vi "Main.vi"(8 "error in (no error)":errorcluster, 11 "Event Registration Refnum":refnum<event-registration>) -> (0 "error out":errorcluster)   [LabVIEW 2023, in "Controller.lvlib"]
uses:
  Controller.lvlib
  Type Def/Module Data.ctl
panel:
  in  "stop":bool
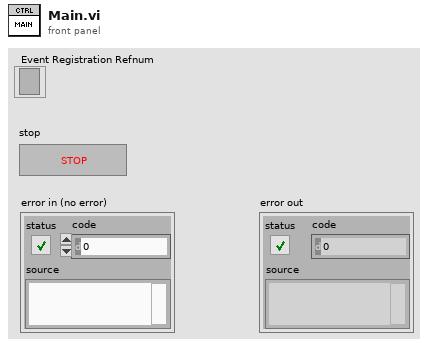
[diagram p1: front panel]
types:
  T1 = typedef "Controller.lvlib/Module Data.ctl" = cluster{"Module Name":string}
  T2 = typedef "Controller.lvlib/Message Data.ctl" = cluster{"Message":string, "Data":variant}
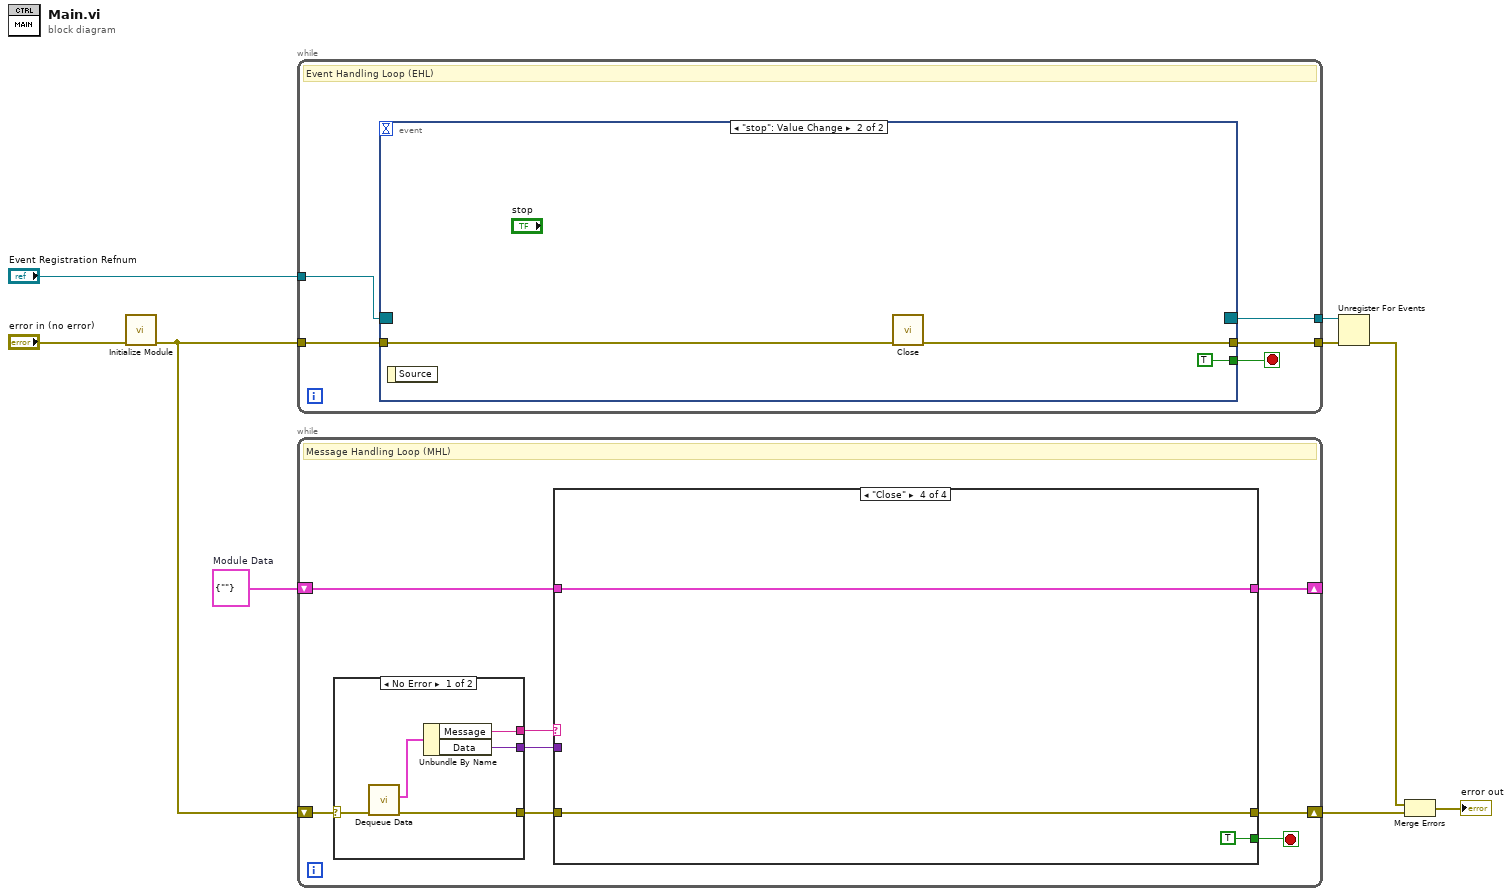
[diagram p0: block diagram]
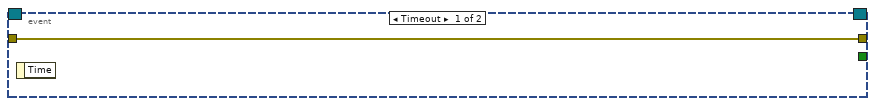
[diagram p2: hidden frame]
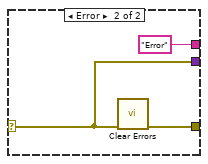
[diagram p3: hidden frame]
diagram:
  w8 = T1 {"Module Name"=""}  # Module Data
  n1 = call "Initialize Module.vi"("error in (no error)"="error in (no error)") -> ("error out"=w7:errorcluster)  [unwired: 10 in]
  n2 = while {
    tunnel: w7 -> [w14]
    tunnel: [w13] -> w4
    tunnel: [w12] -> w2
    tunnel: "Event Registration Refnum" -> [w10]
    stop <- w11 stop-if-true
    # "Event Handling Loop (EHL)"
    n3 = event shown="[1] \"stop\": Value Change" {
      selector: w10 -> [_ _]
      dyn-events: [_ _] -> w12
      timeout: _ -> [_ _]
      tunnel: w14 -> [w15 w18]
      tunnel: [w15 w17] -> w13
      tunnel: [_ TRUE] -> w11
      event Timeout {
        n4 = event-data() -> ()  [unwired: 1 in, 1 out]
      }
      event "stop": Value Change {
        n5 = event-data() -> ()  [unwired: 1 in, 1 out]
        n6 = call "Close.vi"("error in (no error)"=w18) -> ("error out"=w17:errorcluster)  [unwired: 10 in]
      }
    }
  }
  n7 = while {
    shift-right: [w25] -> _
    shift-left: w8 -> [w26]
    shift-right: [w20] -> w6
    shift-left: w7 -> [w24]
    stop <- w19 stop-if-true
    # "Message Handling Loop (MHL)"
    n8 = case shown="No Error" w24 {
      selector: w24 -> [w31 w32]
      tunnel: [w29 "Error" ("Message")] -> w23
      tunnel: [w28 w32] -> w22
      tunnel: [w27 w33] -> w21
      frame No Error {
        n9 = call "Dequeue Data.vi"("error in (no error)"=w31) -> ("error out"=w27:errorcluster, "Message Data"=w30:T2)  [unwired: 9 in]
        n10 = Unbundle By Name(w30) -> ("Message"=w29:string, "Data"=w28:variant)
      }
      frame Error {
        n11 = call <vilib>:"Clear Errors.vi"("error in (no error)"=w32) -> ("error out"=w33:errorcluster)  [unwired: 5 in, 1 out]
      }
    }
    n12 = case shown="\"Close\"" w23 {
      tunnel: w26 -> [w36 w38 w40 w43]
      tunnel: [w36 w38 w40 w43] -> w25
      tunnel: w22 -> [_ _ _ _]
      tunnel: w21 -> [w35 w37 w39 w42]
      tunnel: [w35 w37 w39 w42] -> w20
      tunnel: [_ _ _ TRUE] -> w19
      frame "False", Default {
      }
      frame "Init" {
      }
      frame "Error" {
      }
      frame "Close" {
      }
    }
  }
  n13 = Unregister For Events(event registration refnum=w2, error in=w4) -> (error out=w3:errorcluster)
  n14 = Merge Errors(w3, w6) -> (→"error out":errorcluster)
